vi "Create Test Configuration.vi"() -> (0 "error out":errorcluster, 1 "Names":string[](array[string]), 2 "Line Array":T1[](array[typedef]), 3 "module":refnum<class "Scan Engine configuration.lvclass">, 4 "Channels":refnum<class "TBM channel.lvclass">[](array[class]), 5 "instance identifier":string)   [LabVIEW 2013, in "Scan Engine tests.lvlib"]
doc: "This VI creates the test configuration used in testing. BY default just creates one line with every datatype"
uses:
  Scan Engine tests.lvlib
  configuration/Scan Engine configuration.lvclass
  configuration/Line.ctl
  <vilib>/NI/Tag Bus Module Framework/channel/TBM channel.lvclass
  <vilib>/NI/Tag Bus/tag/Data Type.ctl
  <vilib>/NI/Tag Bus Module Framework/channel/channel classification.ctl
  <vilib>/NI/Configuration Framework/serializable configuration/NISE_CEF_serializable configuration.lvclass
  <vilib>/NI/Tag Bus/tag/tag descriptor.lvclass
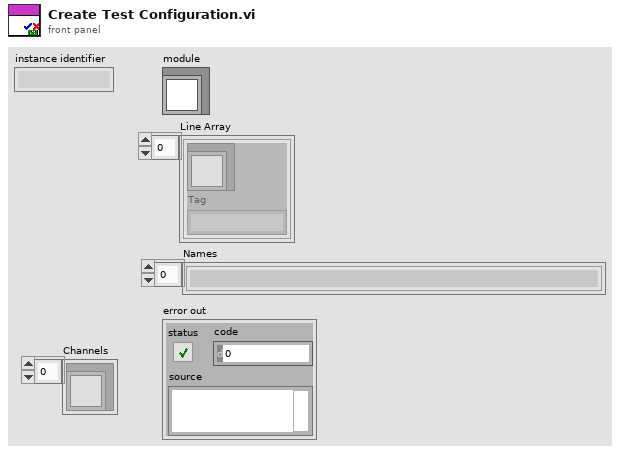
[diagram p1: front panel]
types:
  T1 = typedef "Scan Engine configuration.lvclass/Line.ctl" = cluster{"channel":refnum<class "TBM channel.lvclass">, "Tag":string}
  T2 = typedef "TBM channel.lvclass/channel classification.ctl" = enum16{"input data", "output data", "processing parameter", "processing result"}
  T3 = typedef "tag bus.lvlib/tag descriptor.lvclass/Data Type.ctl" = enum16{"Double", "Single", "I64", "I32", "I16", "I8", "U64", "U32", "U16", "U8", "Boolean", "String", "Array of Double", "Array of Single", "Array of I64", "Array of I32", "Array of I16", "Array of I8", "Array of U64", "Array of U32", "Array of U16", "Array of U8", "Array of Boolean", "Array of String"}
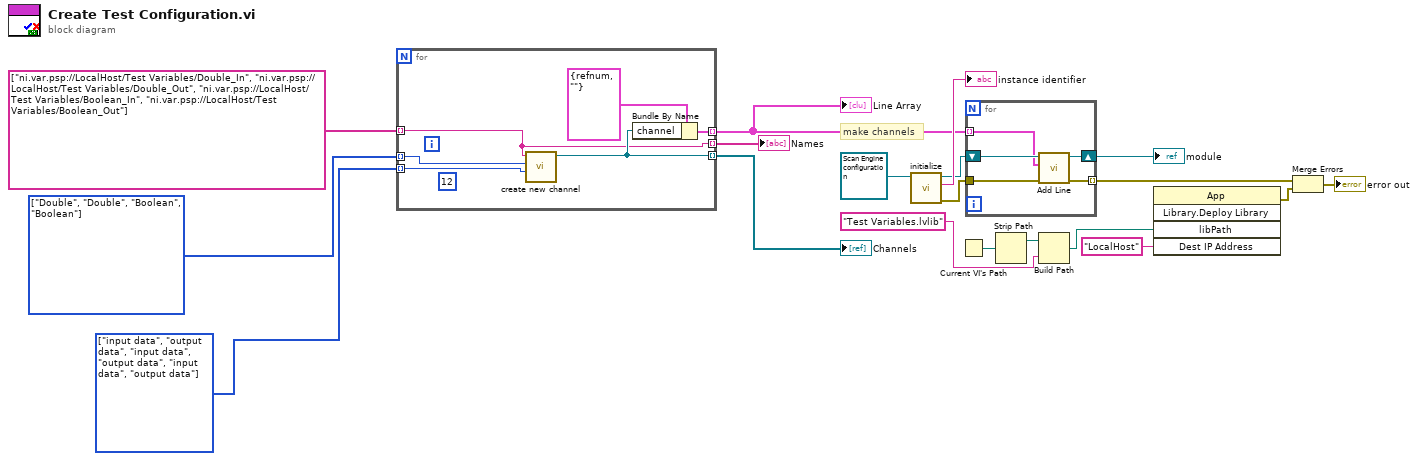
[diagram p0: block diagram]
diagram:
  w1 = T2[] [enum."input data", enum."output data", enum."input data", enum."output data", enum."input data", enum."output data"] items=["input data", "output data", "processing parameter", "processing result"]
  w6 = T3[] [enum."Double", enum."Double", enum."Boolean", enum."Boolean"] items=["Double", "Single", "I64", "I32", "I16", "I8", "U64", "U32", "U16", "U8", "Boolean", "String", "Array of Double", "Array of Single", "Array of I64", "Array of I32", "Array of I16", "Array of I8", "Array of U64", "Array of U32", "Array of U16", "Array of U8", "Array of Boolean", "Array of String"] ("Customize:Properties:supported types")
  # "make channels"
  n1 = for {
    tunnel: w1 -> [w25] mode=indexing
    tunnel: [w22] -> w16 mode=indexing
    tunnel: w6 -> [w24] mode=indexing
    tunnel: [w20] -> w17 mode=indexing
    tunnel: [w21] -> w12 mode=indexing
    tunnel: string[] ["ni.var.psp://LocalHost/Test Variables/Double_In", "ni.var.psp://LocalHost/Test Variables/Double_Out", "ni.var.psp://LocalHost/Test Variables/Boolean_In", "ni.var.psp://LocalHost/Test Variables/Boolean_Out"] ("Names 2") -> [w20] mode=indexing
    (unwired) 12
    n2 = call <vilib>:"create new channel.vi"("channel classification"=w25, "data type"=w24, "channel name"=w20) -> ("channel"=w21:refnum<class "TBM channel.lvclass">)  [unwired: 8 in]
    n3 = Bundle By Name(cluster=T1 {"channel"=refnum, "Tag"=""} ("Line"), "channel"=w21) -> (w22:T1)
  }
  "Names" <- w17
  "Line Array" <- w16
  "Channels" <- w12
  n4 = call <vilib>:"initialize.vi"("configuration in"=refnum<class "Scan Engine configuration.lvclass"> refnum ("tag bus configurable plugin module configuration")) -> ("error out"=w18:errorcluster, "identifier"=→"instance identifier":string, "configuration out"=w13:refnum<class "Scan Engine configuration.lvclass">)  [unwired: 8 in]
  n5 = Current VI's Path() -> (path=w11:path)
  n6 = for {
    tunnel: w16 -> [w26] mode=indexing
    shift-right: [w29] -> w15
    shift-left: w13 -> [w30]
    tunnel: w18 -> [w28]
    tunnel: [w27] -> w4 mode=indexing
    n7 = call "Add Line.vi"("error in"=w28, "Line"=w26, "Scan Engine configuration in"=w30) -> ("error out"=w27:errorcluster, "Scan Engine configuration out"=w29:refnum<class "Scan Engine configuration.lvclass">)  [unwired: 7 in]
  }
  "module" <- w15
  n8 = Strip Path(path=w11) -> (stripped path=w10:path)  [unwired: 1 out]
  n9 = Build Path(base path=w10, name or relative path="Test Variables.lvlib") -> (appended path=w8:path)
  n10 = invoke class="App" method="Library.Deploy Library"("libPath"=w8, "Dest IP Address"="LocalHost" ("Target IPAddress")) -> (error out=w2:errorcluster)  [unwired: 3 in, 4 out]
  n11 = Merge Errors(w4, w2) -> (→"error out":errorcluster)
